vi "Calculate Output.vi"(7 "ADC Readings (input)":T1) -> (8 "Full Output":T2)   [LabVIEW 2017]
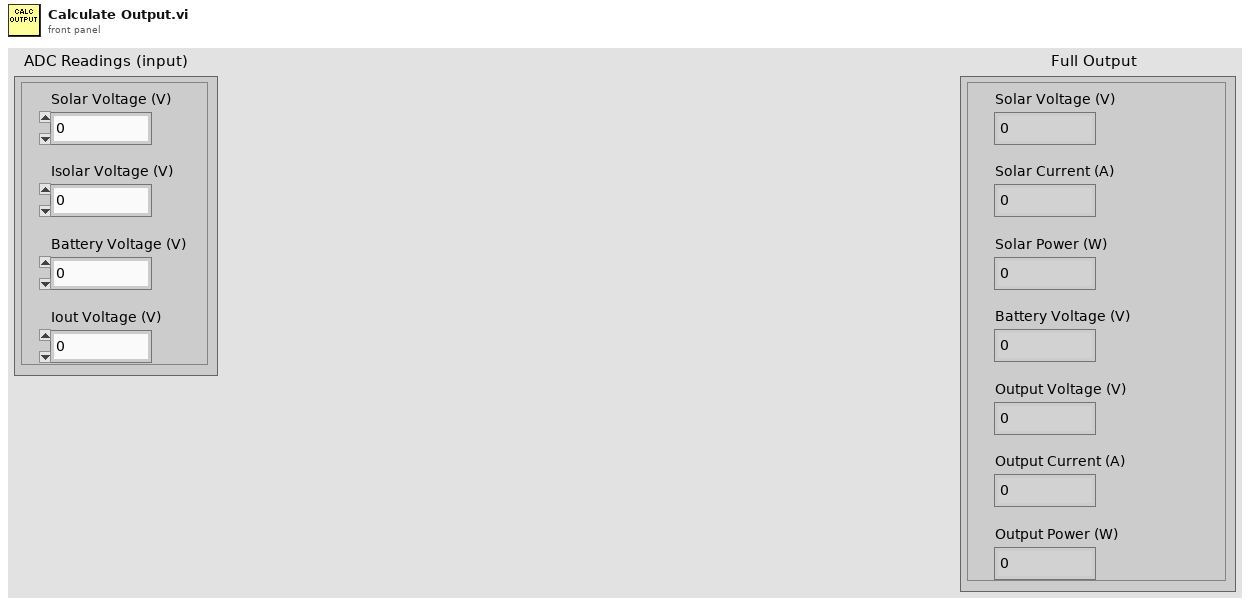
[diagram p1: front panel]
types:
  T1 = cluster{"Solar Voltage (V)":dbl, "Isolar Voltage (V)":dbl, "Battery Voltage (V)":dbl, "Iout Voltage (V)":dbl}
  T2 = cluster{"Solar Voltage (V)":dbl, "Solar Current (A)":dbl, "Solar Power (W)":dbl, "Battery Voltage (V)":dbl, "Output Voltage (V)":dbl, "Output Current (A)":dbl, "Output Power (W)":dbl}
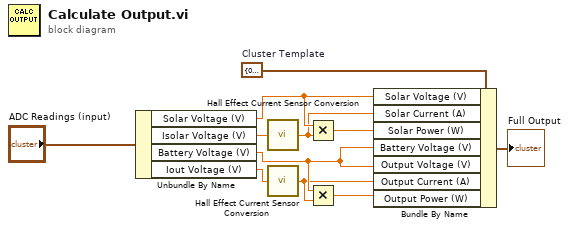
[diagram p0: block diagram]
diagram:
  w10 = T2 {"Solar Voltage (V)"=0.0, "Solar Current (A)"=0.0, "Solar Power (W)"=0.0, "Battery Voltage (V)"=0.0, "Output Voltage (V)"=0.0, "Output Current (A)"=0.0, "Output Power (W)"=0.0}  # Cluster Template
  n1 = Unbundle By Name("ADC Readings (input)") -> ("Solar Voltage (V)"=w7:dbl, "Isolar Voltage (V)"=w5:dbl, "Battery Voltage (V)"=w3:dbl, "Iout Voltage (V)"=w2:dbl)
  n2 = call "Hall Effect Current Sensor Conversion.vi"("Hall Effect Sensor Voltage (V)"=w5) -> ("Hall Effect Sensor Current (A)"=w4:dbl)  [unwired: 8 in]
  n3 = call "Hall Effect Current Sensor Conversion.vi"("Hall Effect Sensor Voltage (V)"=w2) -> ("Hall Effect Sensor Current (A)"=w1:dbl)  [unwired: 8 in]
  n4 = Multiply(x=w7, y=w4) -> (x*y=w8:dbl)
  n5 = Multiply(x=w3, y=w1) -> (x*y=w6:dbl)
  n6 = Bundle By Name(cluster=w10, "Solar Voltage (V)"=w7, "Solar Current (A)"=w4, "Solar Power (W)"=w8, "Battery Voltage (V)"=w3, "Output Voltage (V)"=w3, "Output Current (A)"=w1, "Output Power (W)"=w6) -> (→"Full Output":T2)
